vi "Display Number.vi"(8 "error in (no error)":errorcluster, 9 "Colour":T1 items=["red"=0, "orange"=18, "yellow"=24, "green"=82, "cyan"=127, "blue"=170, "purple"=195, "pink"=220, "white"=254, "black"=255], 10 "Numeric":u16, 11 "Grove 2 RGB LED Matrix In":refnum<class "Grove 2 RGB LED Matrix.lvclass">) -> (0 "error out":errorcluster, 3 "Grove 2 RGB LED Matrix Out":refnum<class "Grove 2 RGB LED Matrix.lvclass">)   [LabVIEW 2020, in "CTI-Peripheral.lvlib" / "Grove 2 RGB LED Matrix.lvclass"]
uses:
  Grove 2 RGB LED Matrix.lvclass
  Data Types/Colors.ctl
  Data Types/MatrixI2CCommand.ctl
  Grove 2 RGB LED Matrix.lvclass/Grove 2 RGB LED Matrix.ctl
  CTI/I2C Connection/I2C Connection.lvclass/I2C Connection.ctl
  CTI/Session/I2C Write Data.vi
  CTI/I2C Connection/I2C Connection.lvclass
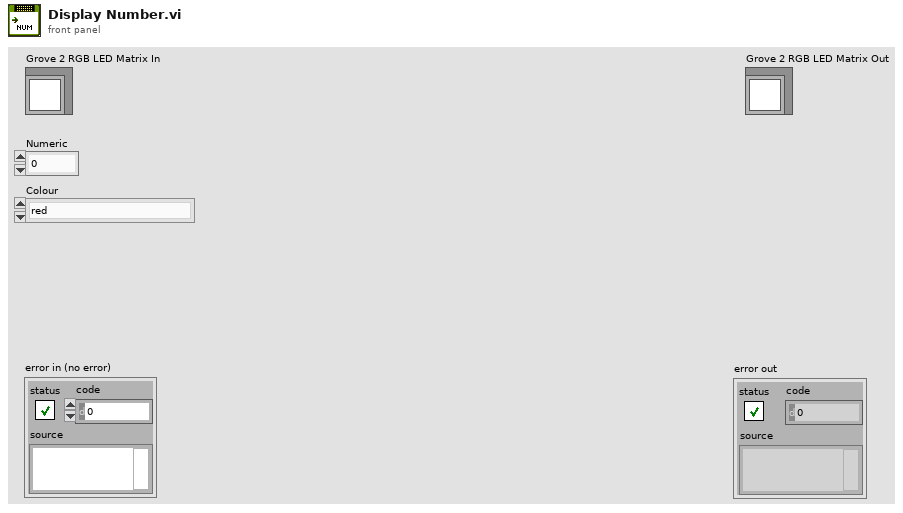
[diagram p1: front panel]
types:
  T1 = typedef "CTI-Peripheral.lvlib/Grove 2 RGB LED Matrix.lvclass/Colors.ctl" = u8
  T2 = typedef "CTI-Peripheral.lvlib/Grove 2 RGB LED Matrix.lvclass/MatrixI2CCommand.ctl" = u8
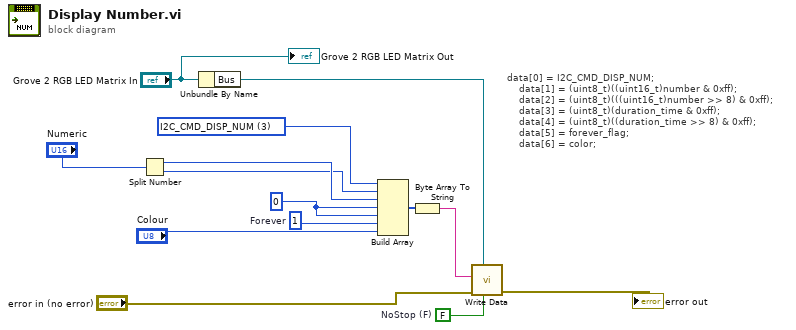
[diagram p0: block diagram]
diagram:
  w5 = u8 0 ("Forever")
  w6 = u8 1  # Forever
  w4 = T2 3 items=["I2C_CMD_GET_DEV_ID"=0, "I2C_CMD_DISP_BAR"=1, "I2C_CMD_DISP_EMOJI"=2, "I2C_CMD_DISP_NUM"=3, "I2C_CMD_DISP_STR"=4, "I2C_CMD_DISP_CUSTOM"=5, "I2C_CMD_DISP_OFF"=6, "I2C_CMD_DISP_ASCII"=7, "I2C_CMD_DISP_FLASH"=8, "I2C_CMD_DISP_COLOR_BAR"=9, "I2C_CMD_DISP_COLOR_WAVE"=10, "I2C_CMD_DISP_COLOR_CLOCKWISE"=11, "I2C_CMD_DISP_COLOR_ANIMATION"=12, "I2C_CMD_DISP_COLOR_BLOCK "=13, "I2C_CMD_STORE_FLASH"=160, "I2C_CMD_DELETE_FLASH"=161, "I2C_CMD_LED_ON"=176, "I2C_CMD_LED_OFF"=177, "I2C_CMD_AUTO_SLEEP_ON"=178, "I2C_CMD_AUTO_SLEEP_OFF"=179, "I2C_CMD_DISP_ROTATE"=180, "I2C_CMD_DISP_OFFSET"=181, "I2C_CMD_SET_ADDR"=192, "I2C_CMD_RST_ADDR"=193, "I2C_CMD_TEST_GET_VER"=226, "I2C_CMD_GET_DEVICE_UID"=241] ("I2C Command")
  w13 = FALSE  # NoStop (F)
  # "data[0] = I2C_CMD_DISP_NUM;\n    data[1] = (uint8_t)((uint16_t)number & 0xff);\n    data[2] = (uint8_t)(((uint16_t)number >> 8) & 0xff);\n    data[3] = (uint8_t)(duration_time & 0xff);\n    data[4] = (uint8_t)((duration_time >> 8) & 0xff);\n    data[5] = forever_flag;\n    data[6] = color;"
  n1 = Split Number(x="Numeric") -> (hi(x)=w2:u8, lo(x)=w1:u8)
  n2 = Unbundle By Name("Grove 2 RGB LED Matrix In") -> ("Bus"=w10:refnum<class "I2C Connection.lvclass">)
  n3 = Build Array(w4, w1, w2, w5, w5, w6, "Colour") -> (w12:T1[])
  n4 = Byte Array To String(unsigned byte array=w12) -> (string=w11:string)
  n5 = call "Write Data.vi"("NoStop (F)"=w13, "I2C Connection"=w10, "error in (no error)"="error in (no error)", "Data"=w11) -> ("error out"=→"error out":errorcluster)  [unwired: 7 in]
  "Grove 2 RGB LED Matrix Out" <- "Grove 2 RGB LED Matrix In"
